vi "picoscopeParseTraceData.vi"(6 "Sample Rate":sgl, 9 "MultiBuffers (Max or non-aggregated)":T2(array[cluster]), 10 "Display Buffer Index":i32, 11 "PicoscopeV2 in":refnum<class "PicoscopeV2.lvclass">) -> (2 "Array":cluster{i32, sgl, "Data":dbl[]}[](array[cluster]), 3 "PicoscopeV2 out":refnum<class "PicoscopeV2.lvclass">)   [LabVIEW 2020, in "PicoscopeV2.lvclass"]
uses:
  PicoscopeV2.lvclass
  PicoscopeV2.lvclass/PicoscopeV2.ctl
panel:
  out "GEECS waveforms info":T1(array[cluster])
  out "scope traces":i16[][](array[numeric])
  out "appended array":waveform(dbl)[](array[waveform])
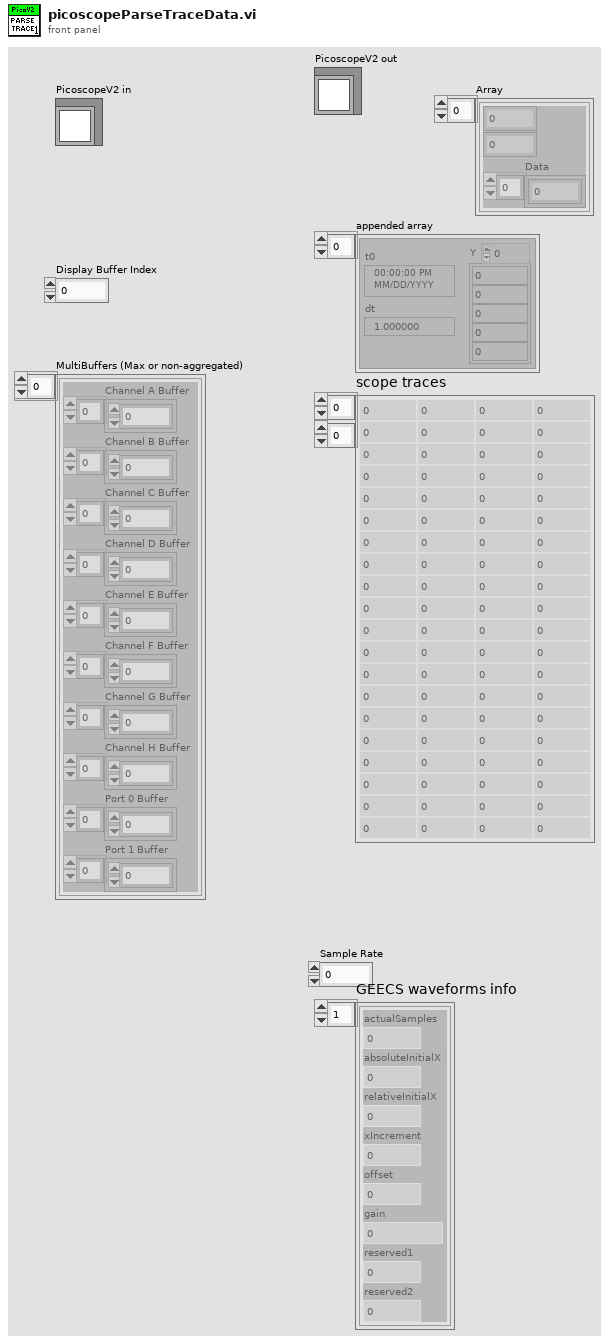
[diagram p1: front panel]
types:
  T1 = cluster{"actualSamples":i32, "absoluteInitialX":dbl, "relativeInitialX":dbl, "xIncrement":dbl, "offset":dbl, "gain":dbl, "reserved1":dbl, "reserved2":dbl}[]
  T2 = cluster{"Channel A Buffer":i16[], "Channel B Buffer":i16[], "Channel C Buffer":i16[], "Channel D Buffer":i16[], "Channel E Buffer":i16[], "Channel F Buffer":i16[], "Channel G Buffer":i16[], "Channel H Buffer":i16[], "Port 0 Buffer":i16[], "Port 1 Buffer":i16[]}[]
  T3 = cluster{"Channel0":string, "Channel1":string, "Channel2":string, "Channel3":string, "Channel4":string, "Channel5":string, "Channel6":string, "Channel7":string}
  T4 = cluster{"NumberofChannels":dbl, "GUInumPoints":i32}
  T5 = typedef "PicoScope5000aAnalogChannelSettings.ctl" = cluster{"Enabled":bool, "Coupling":i16, "Range":u16, "Analogue Offset":sgl, "Bandwidth Limit":u32}
  T6 = cluster{"Channel A Buffer":i16[], "Channel B Buffer":i16[], "Channel C Buffer":i16[], "Channel D Buffer":i16[], "Channel E Buffer":i16[], "Channel F Buffer":i16[], "Channel G Buffer":i16[], "Channel H Buffer":i16[], "Port 0 Buffer":i16[], "Port 1 Buffer":i16[]}
  T7 = typedef "OnOffTypeDef.ctl" = enum16{"off", "on"}
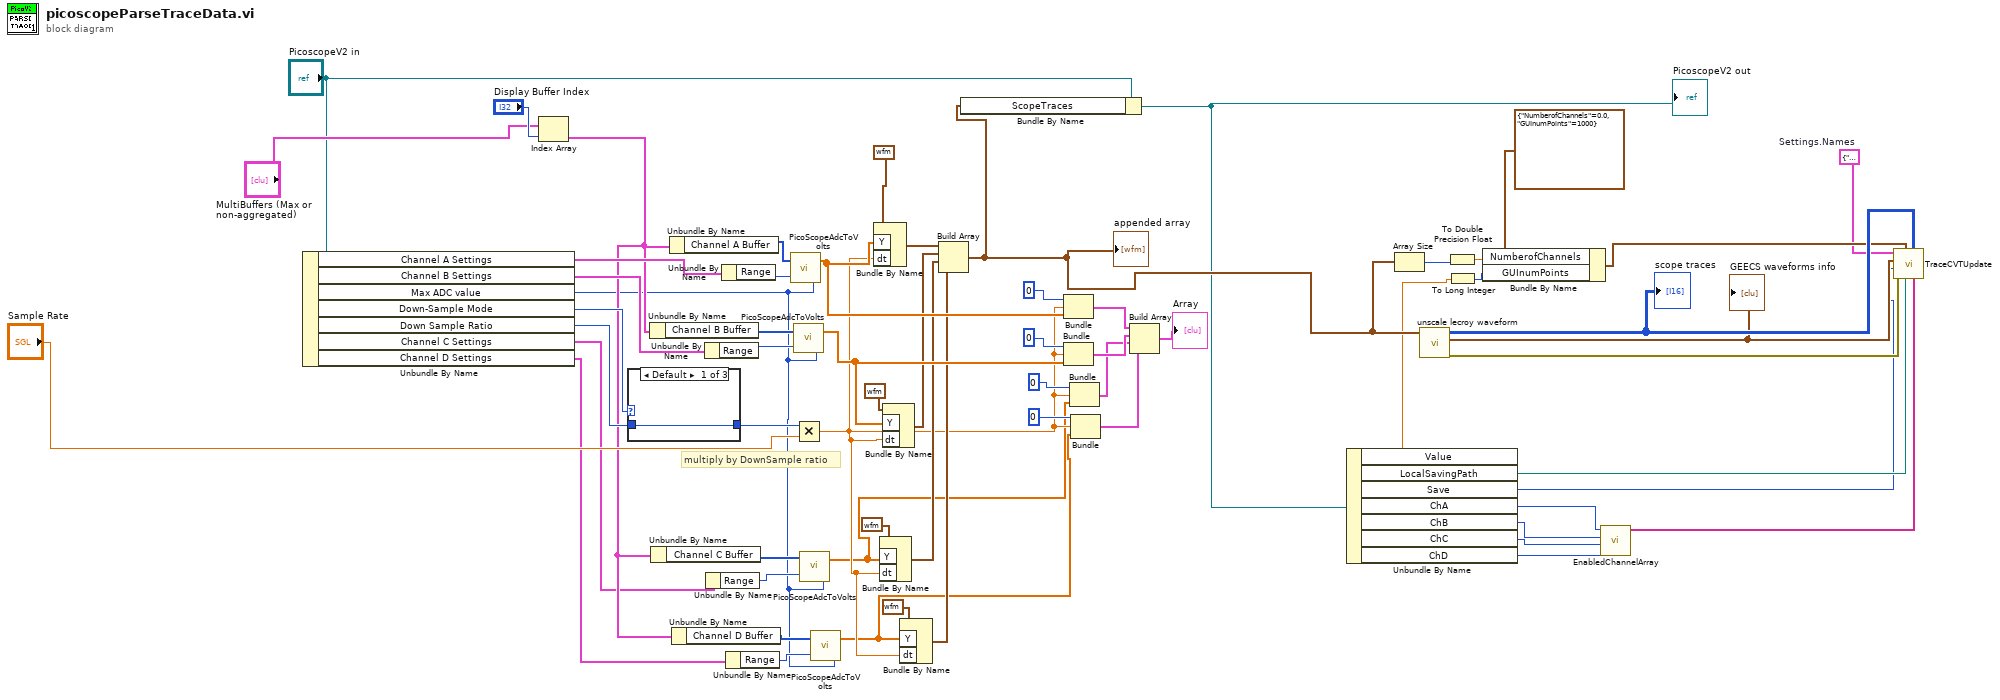
[diagram p0: block diagram]
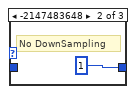
[diagram p2: hidden frame]
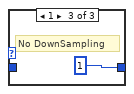
[diagram p3: hidden frame]
diagram:
  w27 = T3 {"Channel0"="Channel0", "Channel1"="Channel1", "Channel2"="Channel2", "Channel3"="Channel3", "Channel4"="", "Channel5"="", "Channel6"="", "Channel7"=""}  # Settings.Names
  # "multiply by DownSample ratio"
  n1 = Unbundle By Name("PicoscopeV2 in") -> ("Channel A Settings"=w49:T5, "Channel B Settings"=w50:T5, "Max ADC value"=w12:i16, "Down-Sample Mode"=w61:u32, "Down Sample Ratio"=w62:u64, "Channel C Settings"=w15:T5, "Channel D Settings"=w14:T5)
  n2 = Index Array(array="MultiBuffers (Max or non-aggregated)", index="Display Buffer Index") -> (element=w16:T6)
  n3 = case shown="Default" w61 {
    tunnel: [w63 u64 1 ("Down Sample Ratio") u64 1 ("Down Sample Ratio")] -> w13
    tunnel: w62 -> [w63 _ _]
    frame Default {
    }
    frame -2147483648 {
      # "No DownSampling"
    }
    frame 1 {
      # "No DownSampling"
    }
  }
  n4 = Unbundle By Name(w16) -> ("Channel B Buffer"=w54:i16[])
  n5 = Unbundle By Name(w16) -> ("Channel C Buffer"=w17:i16[])
  n6 = Unbundle By Name(w16) -> ("Channel A Buffer"=w58:i16[])
  n7 = Unbundle By Name(w16) -> ("Channel D Buffer"=w18:i16[])
  n8 = Unbundle By Name(w50) -> ("Range"=w60:u16)
  n9 = Unbundle By Name(w15) -> ("Range"=w20:u16)
  n10 = Unbundle By Name(w49) -> ("Range"=w52:u16)
  n11 = Unbundle By Name(w14) -> ("Range"=w19:u16)
  n12 = call "PicoScopeAdcToVolts.vi"("Max_adc"=w12, "Range Index"=w52, "Data"=w58) -> ("Data"=w43:dbl[])
  n13 = call "PicoScopeAdcToVolts.vi"("Max_adc"=w12, "Range Index"=w60, "Data"=w54) -> ("Data"=w46:dbl[])
  n14 = Multiply(x=w13, y="Sample Rate") -> (x*y=w5:sgl)
  n15 = call "PicoScopeAdcToVolts.vi"("Max_adc"=w12, "Range Index"=w20, "Data"=w17) -> ("Data"=w4:dbl[])
  n16 = call "PicoScopeAdcToVolts.vi"("Max_adc"=w12, "Range Index"=w19, "Data"=w18) -> ("Data"=w3:dbl[])
  n17 = Bundle By Name(cluster=waveform(dbl) {"t0"=timestamp(0 s since 1904-01-01), "dt"=1.0, "Y"=[]} ("waveform"), "Y"=w43, "dt"=w5) -> (w42:waveform(dbl))
  n18 = Bundle By Name(cluster=waveform(dbl) {"t0"=timestamp(0 s since 1904-01-01), "dt"=1.0, "Y"=[]} ("waveform"), "Y"=w4, "dt"=w5) -> (w9:waveform(dbl))
  n19 = Bundle By Name(cluster=waveform(dbl) {"t0"=timestamp(0 s since 1904-01-01), "dt"=1.0, "Y"=[]} ("waveform"), "Y"=w46, "dt"=w5) -> (w41:waveform(dbl))
  n20 = Bundle By Name(cluster=waveform(dbl) {"t0"=timestamp(0 s since 1904-01-01), "dt"=1.0, "Y"=[]} ("waveform"), "Y"=w3, "dt"=w5) -> (w8:waveform(dbl))
  n21 = Build Array(w42, w41, w9, w8) -> (w39:waveform(dbl)[])
  "appended array" <- w39
  n22 = Bundle By Name(cluster="PicoscopeV2 in", "ScopeTraces"=w39) -> (w38:refnum<class "PicoscopeV2.lvclass">)
  "PicoscopeV2 out" <- w38
  n23 = Bundle(0, w5, "Data"=w43) -> (w55:cluster{i32, sgl, "Data":dbl[]})  [unwired: 1 in]
  n24 = Bundle(0, w5, "Data"=w46) -> (w56:cluster{i32, sgl, "Data":dbl[]})  [unwired: 1 in]
  n25 = Bundle(0, w5, "Data"=w4) -> (w2:cluster{i32, sgl, "Data":dbl[]})  [unwired: 1 in]
  n26 = Bundle(0, w5, "Data"=w3) -> (w1:cluster{i32, sgl, "Data":dbl[]})  [unwired: 1 in]
  n27 = Build Array(w55, w56, w2, w1) -> (→"Array":cluster{i32, sgl, "Data":dbl[]}[])
  n28 = Unbundle By Name(w38) -> ("Value"=w35:dbl, "LocalSavingPath"=w28:path, "Save"=w26:T7, "ChA"=w25:T7, "ChB"=w24:T7, "ChC"=w22:T7, "ChD"=w21:T7)
  n29 = Array Size(array=w39) -> (size(s)=w33:i32)
  n30 = call "unscale lecroy waveform.vi"("Waveforms"=w39) -> ("Error out"=w29:errorcluster, "GEECS waveforms info"=w30:T1, "scope traces"=w32:i16[][])  [unwired: 8 in]
  "scope traces" <- w32
  "GEECS waveforms info" <- w30
  n31 = To Double Precision Float(number=w33) -> (double precision float=w34:dbl)
  n32 = To Long Integer(number=w35) -> (32bit integer=w36:i32)
  n33 = Bundle By Name(cluster=T4 {"NumberofChannels"=0.0, "GUInumPoints"=1000}, "NumberofChannels"=w34, "GUInumPoints"=w36) -> (w31:T4)
  n34 = call "EnabledChannelArray.vi"("Channel3"=w21, "Channel2"=w22, "Channel1"=w24, "Channel0"=w25) -> ("EnabledChannels"=w23:string[])  [unwired: 7 in]
  n35 = call "TraceCVTUpdate.vi"("Channels"=w23, "wfm"=w32, "Settings.LocalSavingPath"=w28, "TraceGUI-Info"=w31, "error in (no error)"=w29, "Save"=w26, "wfm info"=w30, "Settings.Names"=w27) -> ()  [unwired: 1 in, 3 out]
